vi "Select_Inspection_UI.vi"(8 "error in (no error)":errorcluster, 11 "ZenGage v3.0 UI in":refnum<class "ZenGage v3.0 UI.lvclass">) -> (0 "error out":errorcluster, 3 "ZenGage v3.0 UI out":refnum<class "ZenGage v3.0 UI.lvclass">)   [LabVIEW 2015, in "ZenGage v3.0 UI.lvclass"]
uses:
  ZenGage v3.0 UI.lvclass
  ZenGage v3.0 UI.lvclass/ZenGage v3.0 UI.ctl
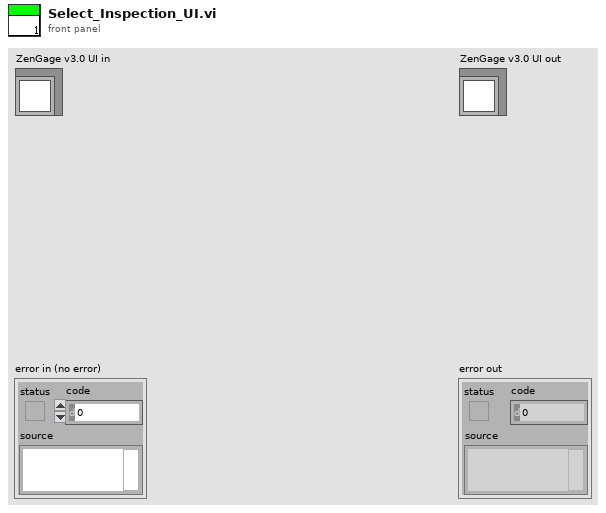
[diagram p1: front panel]
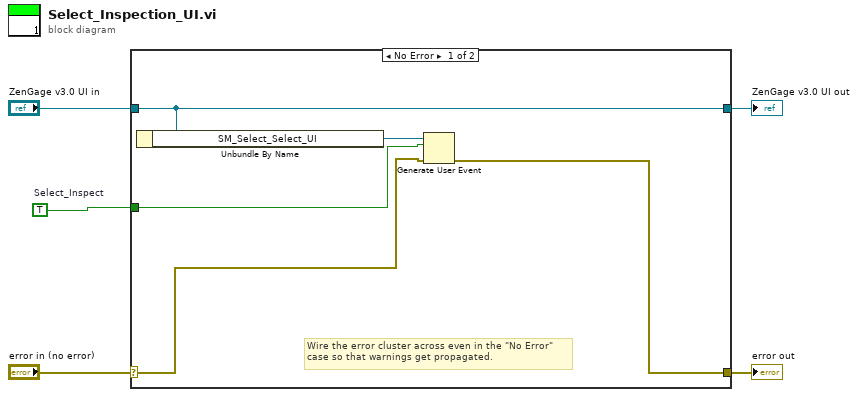
[diagram p0: block diagram]
diagram:
  w1 = TRUE  # Select_Inspect
  n1 = case shown="No Error" "error in (no error)" {
    selector: "error in (no error)" -> [w7 w12]
    tunnel: [w6 w12] -> w4
    tunnel: [w10 w11] -> w2
    tunnel: "ZenGage v3.0 UI in" -> [w10 w11]
    tunnel: w1 -> [w8 _]
    frame No Error {
      # "Wire the error cluster across even in the \"No Error\"\ncase so that warnings get propagated."
      n2 = Unbundle By Name(w10) -> ("SM_Select_Select_UI"=w9:refnum<user-event>)
      n3 = Generate User Event(user event=w9, event data cluster=w8, error in=w7) -> (error out=w6:errorcluster)  [unwired: 1 in, 1 out]
    }
    frame Error {
    }
  }
  "error out" <- w4
  "ZenGage v3.0 UI out" <- w2
